vi "Colortable-set.vi"(7 "Invert":bool, 10 "Color table in":dbl[](array[numeric]), 11 "Select CTable 2":T1 items=["blue color", "infrared color", "RB black", "Unchanged", "Purple", "Yellow", "Green", "Red", "'B-W LINEAR'", " 'BLUE-WHITE'", "'GRN-RED-BLU-WHT'", "'RED TEMPERATURE'", "'BLUE-GREEN-RED-YELLOW'", "'STD GAMMA-II'", "'PRISM'", "'RED-PURPLE'", "'GREEN-WHITE LINEAR'", "'GRN-WHT EXPONENTIAL'", "'GREEN-PINK'", "'BLUE-RED'", "'16 LEVEL'", "'RAINBOW'", "'STEPS'", "'STERN SPECIAL'", "'Haze'", "'Blue - Pastel - Red'", "'Pastels'", "'Hue Sat Lightness 1'", "'Hue Sat Lightness 2'", "'Hue Sat Value 1'", "'Hue Sat Value 2'", "'Purple-Red + Stripes'", "'Beach'", "'Mac Style'", "'Eos A'", "'Eos B'", "'Hardcandy'", "'Nature'", "'Ocean'", "'Peppermint'", "'Plasma'", "'Blue-Red'", "'Rainbow'", "'Blue Waves'", "'Volcano'", "'Waves'", "'Rainbow18'", "'Rainbow + white'", "'Rainbow + black'", "'CB-Accent'", "'CB-Dark2'", "'CB-Paired'", "'CB-Pastel1'", "'CB-Pastel2'", "'CB-Set1'", "'CB-Set2'", "'CB-Set3'", "'CB-Blues'", "'CB-BuGn'", "'CB-BuPu'", "'CB-GnBu'", "'CB-Greens'", "'CB-Greys'", "'CB-Oranges'", "'CB-OrRd'", "'CB-PuBu'", "'CB-PuBuGn'", "'CB-PuRd'", "'CB-Purples'", "'CB-RdPu'", "'CB-Reds'", "'CB-YlGn'", "'CB-YlGnBu'", "'CB-YlOrBr'", "'CB-BrBG'", "'CB-PiYG'", "'CB-PRGn'", "'CB-PuOr'", "'CB-RdBu'", "'CB-RdGy'", "'CB-RdYlBu'", "'CB-RdYlG'", "'CB-Spectra'"]) -> (3 "Color table out":u32[](array[numeric]))   [LabVIEW 2019]
uses:
  <userlib>/_Color/Color Table .ctl
panel:
  out "CT index 2":i32 format="%.0x"
  in  "Color Box":u32(colorbox)
  out "CT index":i32
  out "size(s) 2":i32[](array[numeric])
  out "CT name":string
  out "Color tables all 2":u32[][](array[colorbox])
  out "Strings []":string[](array[string])=["blue color", "infrared color", "weird c-table", "Unchanged", "Yellowish", "Green", "Yellow", "B/W", "'B-W LINEAR'", " 'BLUE-WHITE'", "'GRN-RED-BLU-WHT'", "'RED TEMPERATURE'", "'BLUE-GREEN-RED-YELLOW'", "'STD GAMMA-II'", "'PRISM'", "'RED-PURPLE'", "'GREEN-WHITE LINEAR'", "'GRN-WHT EXPONENTIAL'", "'GREEN-PINK'", "'BLUE-RED'", "'16 LEVEL'", "'RAINBOW'", "'STEPS'", "'STERN SPECIAL'", "'Haze'", "'Blue - Pastel - Red'", "'Pastels'", "'Hue Sat Lightness 1'", "'Hue Sat Lightness 2'", "'Hue Sat Value 1'", "'Hue Sat Value 2'", "'Purple-Red + Stripes'", "'Beach'", "'Mac Style'", "'Eos A'", "'Eos B'", "'Hardcandy'", "'Nature'", "'Ocean'", "'Peppermint'", "'Plasma'", "'Blue-Red'", "'Rainbow'", "'Blue Waves'", "'Volcano'", "'Waves'", "'Rainbow18'", "'Rainbow + white'", "'Rainbow + black'", "'CB-Accent'", "'CB-Dark2'", "'CB-Paired'", "'CB-Pastel1'", "'CB-Pastel2'", "'CB-Set1'", "'CB-Set2'", "'CB-Set3'", "'CB-Blues'", "'CB-BuGn'", "'CB-BuPu'", "'CB-GnBu'", "'CB-Greens'", "'CB-Greys'", "'CB-Oranges'", "'CB-OrRd'", "'CB-PuBu'", "'CB-PuBuGn'", "'CB-PuRd'", "'CB-Purples'", "'CB-RdPu'", "'CB-Reds'", "'CB-YlGn'", "'CB-YlGnBu'", "'CB-YlOrBr'", "'CB-BrBG'", "'CB-PiYG'", "'CB-PRGn'", "'CB-PuOr'", "'CB-RdBu'", "'CB-RdGy'", "'CB-RdYlBu'", "'CB-RdYlG'", "'CB-Spectra'"]
  in  "Color tables all":u32[][](array[colorbox])=array75x256[19200 elements]
  in  "color table names":string[](array[string])=["'B-W LINEAR'", " 'BLUE-WHITE'", "'GRN-RED-BLU-WHT'", "'RED TEMPERATURE'", "'BLUE-GREEN-RED-YELLOW'", "'STD GAMMA-II'", "'PRISM'", "'RED-PURPLE'", "'GREEN-WHITE LINEAR'", "'GRN-WHT EXPONENTIAL'", "'GREEN-PINK'", "'BLUE-RED'", "'16 LEVEL'", "'RAINBOW'", "'STEPS'", "'STERN SPECIAL'", "'Haze'", "'Blue - Pastel - Red'", "'Pastels'", "'Hue Sat Lightness 1'", "'Hue Sat Lightness 2'", "'Hue Sat Value 1'", "'Hue Sat Value 2'", "'Purple-Red + Stripes'", "'Beach'", "'Mac Style'", "'Eos A'", "'Eos B'", "'Hardcandy'", "'Nature'", "'Ocean'", "'Peppermint'", "'Plasma'", "'Blue-Red'", "'Rainbow'", "'Blue Waves'", "'Volcano'", "'Waves'", "'Rainbow18'", "'Rainbow + white'", "'Rainbow + black'", "'CB-Accent'", "'CB-Dark2'", "'CB-Paired'", "'CB-Pastel1'", "'CB-Pastel2'", "'CB-Set1'", "'CB-Set2'", "'CB-Set3'", "'CB-Blues'", "'CB-BuGn'", "'CB-BuPu'", "'CB-GnBu'", "'CB-Greens'", "'CB-Greys'", "'CB-Oranges'", "'CB-OrRd'", "'CB-PuBu'", "'CB-PuBuGn'", "'CB-PuRd'", "'CB-Purples'", "'CB-RdPu'", "'CB-Reds'", "'CB-YlGn'", "'CB-YlGnBu'", "'CB-YlOrBr'", "'CB-BrBG'", "'CB-PiYG'", "'CB-PRGn'", "'CB-PuOr'", "'CB-RdBu'", "'CB-RdGy'", "'CB-RdYlBu'", "'CB-RdYlG'", "'CB-Spectra'"]
  out "size(s)":i32
  out "CT array":u32[](array[colorbox])
  out "Color table out 2":dbl[](array[numeric])
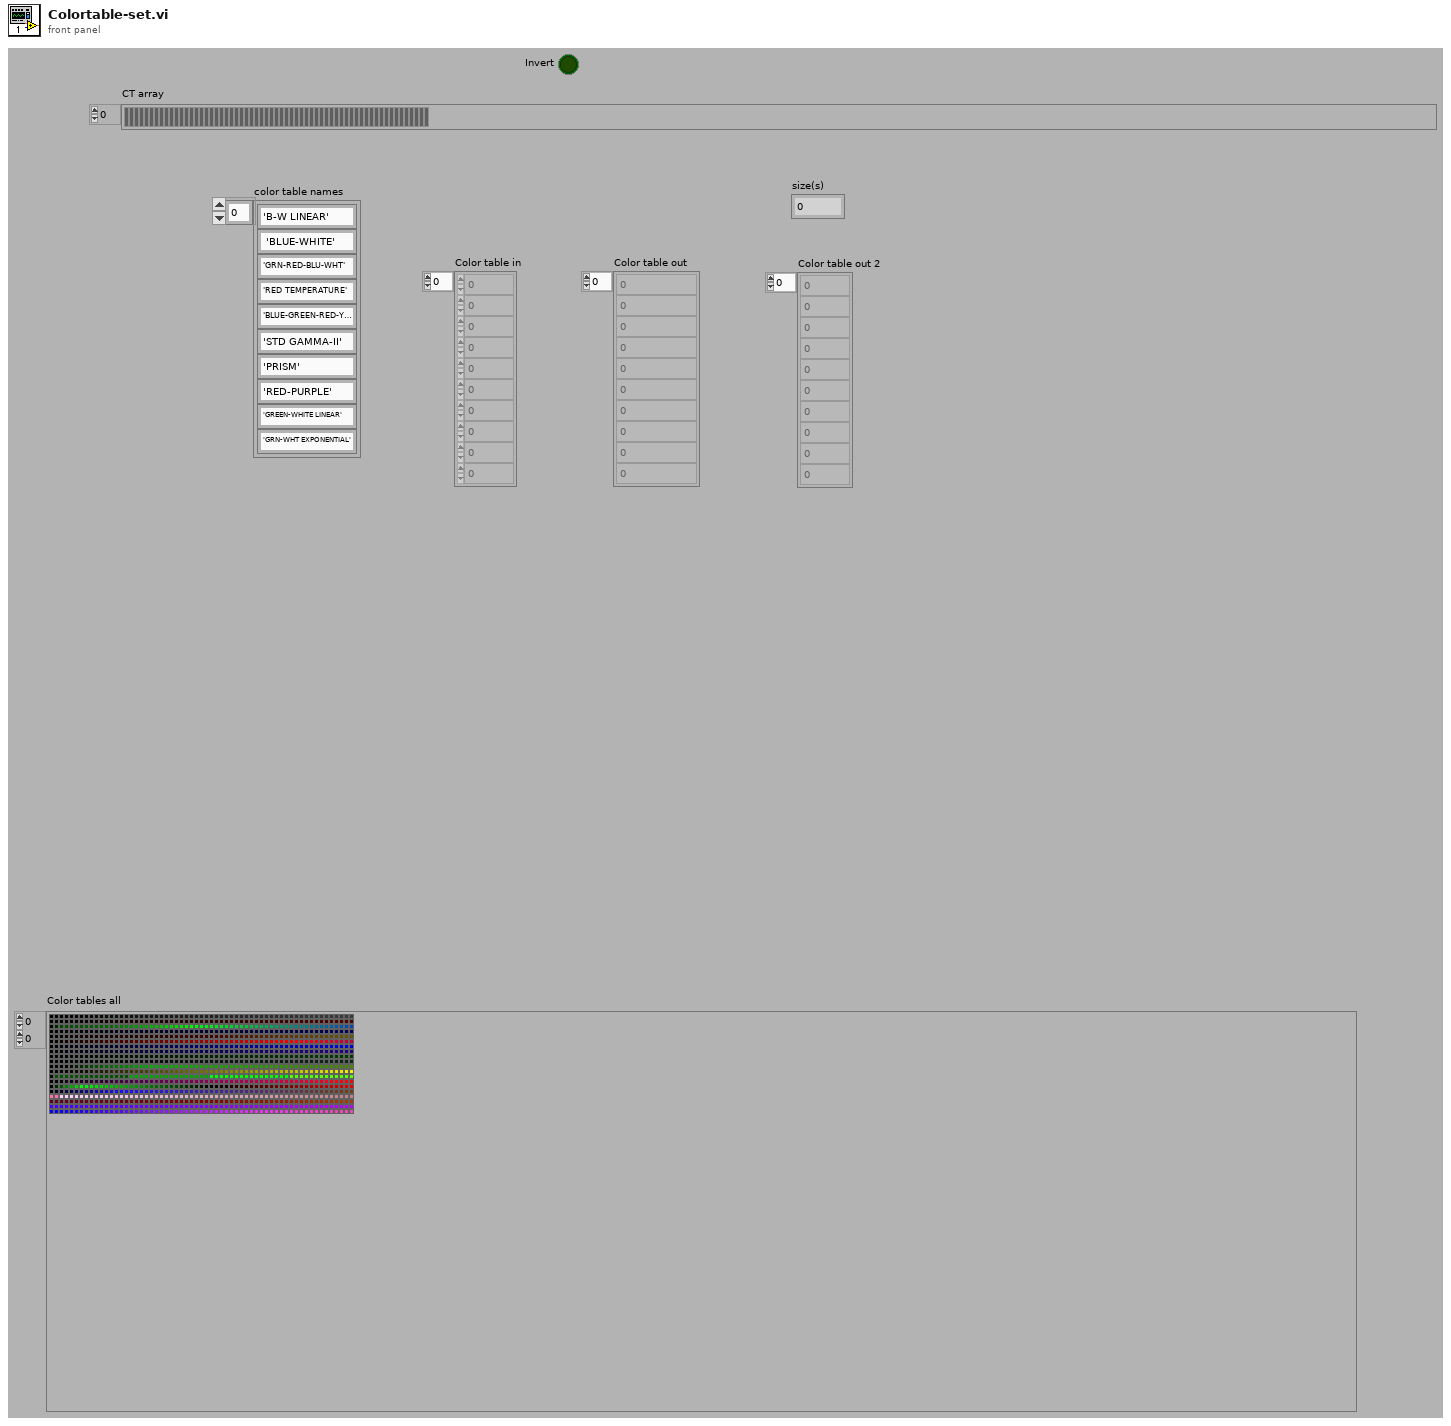
[diagram p1: front panel]
types:
  T1 = typedef "Color Table .ctl" = u16
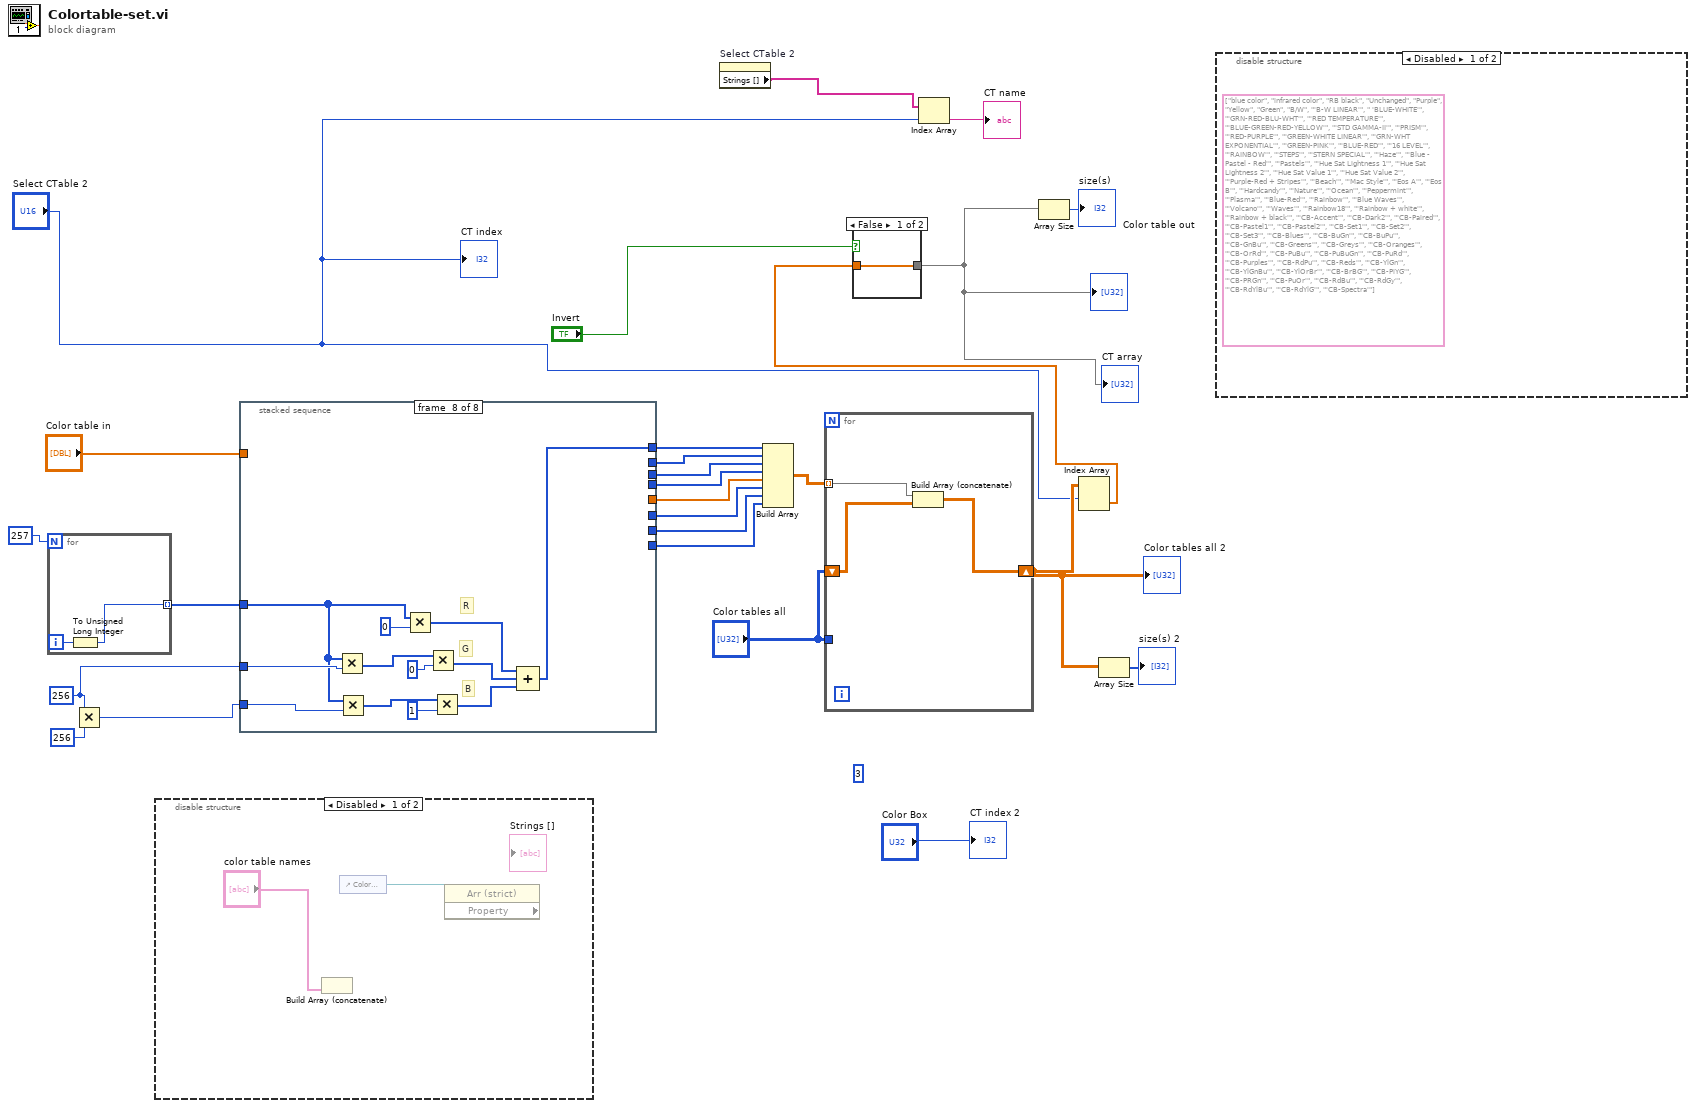
[diagram p0: block diagram]
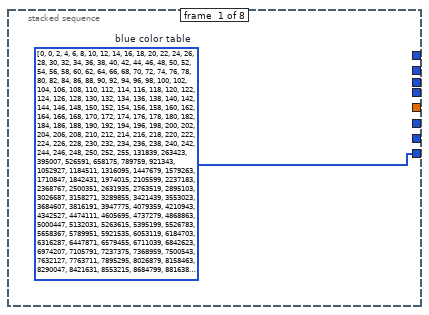
[diagram p3: hidden frame]
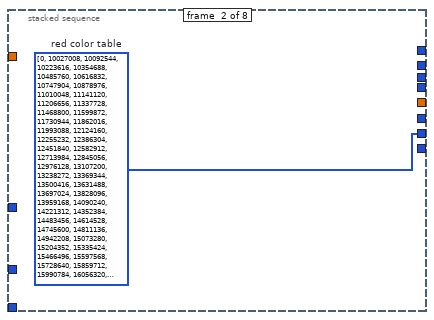
[diagram p4: hidden frame]
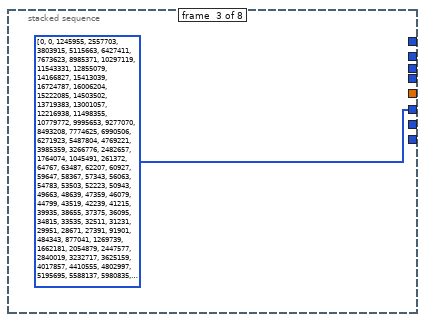
[diagram p5: hidden frame]
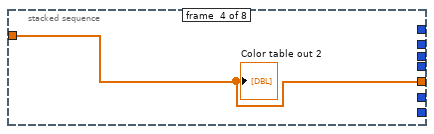
[diagram p6: hidden frame]
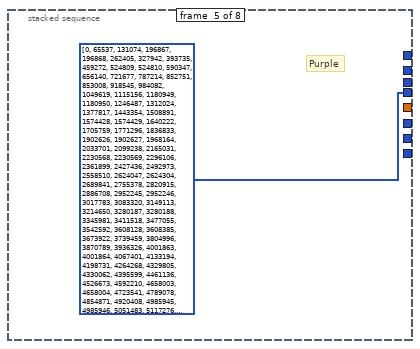
[diagram p7: hidden frame]
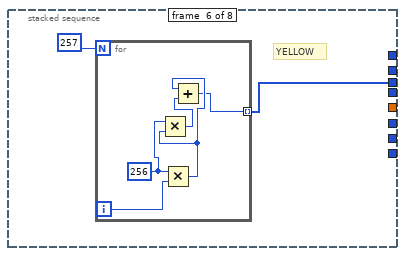
[diagram p8: hidden frame]
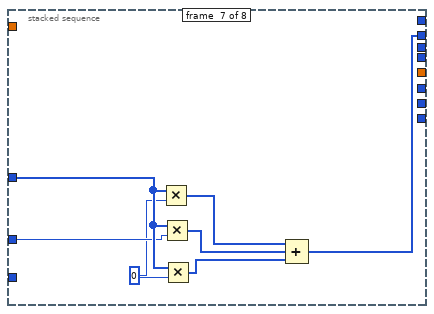
[diagram p9: hidden frame]
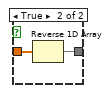
[diagram p11: hidden frame]
diagram:
  w5 = u32 256 ("x")
  (unwired) 3
  n1 = for {
    N: u32 257 -> [_]
    tunnel: [w27] -> w7 mode=indexing
    i -> [w28]
    n2 = To Unsigned Long Integer(number=w28) -> (unsigned 32bit integer=w27:u32)
  }
  n3 = Multiply(x=w5, y=u32 256 ("x")) -> (x*y=w4:u32)
  n4 = disable-structure shown="Disabled" {
    frame Disabled {
      n5 = Build Array (concatenate)("color table names") -> (w31:string[], w32:string[])
      n6 = control-ref of="Color table in"() -> (w30:refnum<vi>)
      n7 = property class="Arr (strict)" props=[](reference=w30) -> ()  [unwired: 1 in, 3 out]
    }
    frame Enabled {
    }
  }
  n8 = stacked-sequence {
    tunnel: "Color table in" -> [_ _ _ w37 _ _ _ _]
    tunnel: [_ _ _ _ u32[] [0, 65537, 131074, 196867, 196868, 262405, 327942, 393735, 459272, 524809, 524810, 590347, 656140, 721677, 787214, 852751, 853008, 918545, 984082, 1049619, 1115156, 1180949, 1180950, 1246487, 1312024, 1377817, 1443354, 1508891, 1574428, 1574429, 1640222, 1705759, 1771296, 1836833, 1902626, 1902627, 1968164, 2033701, 2099238, 2165031, 2230568, 2230569, 2296106, 2361899, 2427436, 2492973, 2558510, 2624047, 2624304, 2689841, 2755378, 2820915, 2886708, 2952245, 2952246, 3017783, 3083320, 3149113, 3214650, 3280187, 3280188, 3345981, 3411518, 3477055, 3542592, 3608128, 3608385, 3673922, 3739459, 3804996, 3870789, 3936326, 4001863, 4001864, 4067401, 4133194, 4198731, 4264268, 4329805, 4330062, 4395599, 4461136, 4526673, 4592210, 4658003, 4658004, 4723541, 4789078, 4854871, 4920408, 4985945, 4985946, 5051483, 5117276, 5182813, 5248350, 5313887, 5379680, 5379681, 5445218, 5510755, 5576292, 5642085, 5707622, 5707623, 5773160, 5838953, 5904490, 5970027, 6035564, 6035565, 6101358, 6166895, 6232432, 6297969, 6363762, 6363763, 6429300, 6494837, 6560374, 6626167, 6691704, 6757241, 6757242, 6823035, 6888572, 6954109, 7019646, 7085183, 7085440, 7150977, 7216514, 7282051, 7347588, 7413381, 7413382, 7478919, 7544456, 7610249, 7675786, 7741323, 7806860, 7806861, 7872654, 7938191, 8003728, 8069265, 8135058, 8135059, 8200596, 8266133, 8331670, 8397463, 8463000, 8463001, 8528538, 8594331, 8659868, 8725405, 8790942, 8790943, 8856736, 8922273, 8987810, 9053347, 9119140, 9184677, 9184678, 9250215, 9315752, 9381545, 9447082, 9512619, 9512620, 9578413, 9643950, 9709487, 9775024, 9840561, 9840818, 9906355, 9971892, 10037429, 10103222, 10168759, 10168760, 10234297, 10299834, 10365627, 10431164, 10496701, 10562238, 10562495, 10628031, 10693568, 10759105, 10824642, 10890435, 10890436, 10955973, 11021510, 11087303, 11152840, 11218377, 11218378, 11283915, 11349708, 11415245, 11480782, 11546319, 11546576, 11612113, 11677650, 11743187, 11808724, 11874517, 11940054, 11940055, 12005592, 12071385, 12136922, 12202459, 12267996, 12267997, 12333790, 12399327, 12464864, 12530401, 12596194, 12596195, 12661732, 12727269, 12792806, 12858599, 12924136, 12989673, 12989674, 13055467, 13121004, 13186541, 13252078, 13317615, 13317872, 13383409, 13448946, 13514483, 13580276, 13645813, 13645814, 13711351, 13776888, 13842681, 13908218, 13973755, 13973756, 14039549, 14105086] ("Clrtbl out") _ _ _] -> w22
    tunnel: [_ _ _ w37 _ _ _ _] -> w21
    tunnel: [_ _ u32[] [0, 0, 1245955, 2557703, 3803915, 5115663, 6427411, 7673623, 8985371, 10297119, 11543331, 12855079, 14166827, 15413039, 16724787, 16006204, 15222085, 14503502, 13719383, 13001057, 12216938, 11498355, 10779772, 9995653, 9277070, 8493208, 7774625, 6990506, 6271923, 5487804, 4769221, 3985359, 3266776, 2482657, 1764074, 1045491, 261372, 64767, 63487, 62207, 60927, 59647, 58367, 57343, 56063, 54783, 53503, 52223, 50943, 49663, 48639, 47359, 46079, 44799, 43519, 42239, 41215, 39935, 38655, 37375, 36095, 34815, 33535, 32511, 31231, 29951, 28671, 27391, 91901, 484343, 877041, 1269739, 1662181, 2054879, 2447577, 2840019, 3232717, 3625159, 4017857, 4410555, 4802997, 5195695, 5588137, 5980835, 6373533, 6765975, 7158673, 7551115, 7943813, 8336511, 8728953, 9121651, 9514093, 9906791, 10299489, 10626396, 11019094, 11411792, 11804234, 12196932, 12589374, 12982072, 13374770, 13767212, 14159910, 14552352, 14945050, 15337748, 15730190, 16122888, 16515330, 16712192, 16713216, 16713984, 16715008, 16716032, 16717056, 16718080, 16718848, 16719872, 16720896, 16721920, 16722944, 16723712, 16724736, 16725760, 16726784, 16727808, 16728576, 16729600, 16730624, 16731648, 16732672, 16733440, 16734464, 16735488, 16736512, 16737280, 16738304, 16739328, 16740352, 16741376, 16742144, 16743168, 16744192, 16745216, 16746240, 16747008, 16748032, 16749056, 16750080, 16751104, 16751872, 16752896, 16753920, 16754944, 16755968, 16756736, 16757760, 16758784, 16759808, 16760832, 16761600, 16762624, 16763648, 16370944, 15912448, 15454208, 14995712, 14471936, 14013440, 13554944, 13096704, 12572672, 12114432, 11655936, 11197696, 10739200, 10215424, 9756928, 9298432, 8840192, 8316160, 7857920, 7399424, 6941184, 6417152, 5958912, 5500416, 5041920, 4518144, 4059648, 3601408, 3142912, 2619136, 2160640, 1702400, 1243904, 720128, 261632, 261890, 589574, 982794, 1310478, 1703699, 2031383, 2424603, 2752287, 3145507, 3473191, 3866411, 4194095, 4587316, 4915000, 5308220, 5635904, 6029124, 6356808, 6750028, 7077712, 7470933, 7798617, 8191837, 8519521, 8912741, 9240425, 9633645, 9961329, 10354550, 10682234, 11075454, 11403138, 11796358, 12124042, 12517262, 12844946, 13238167, 13434777, 13434777, 13434777, 13434777, 13434777, 13434777, 13434777, 13434777, 13434777, 13434777, 13434777, 13434777, 13434777, 13434777, 13434777, 13434777, 13434777, 13434777, 16777215] ("Write Attribute") _ _ _ _ _] -> w20
    tunnel: [_ w35 _ _ _ _ _ _] -> w19
    tunnel: [w34 _ _ _ _ _ _ _] -> w18
    tunnel: [_ _ _ _ _ w39 _ _] -> w11
    tunnel: [_ _ _ _ _ _ w50 _] -> w10
    tunnel: w7 -> [_ _ _ _ _ _ w49 w59]
    tunnel: w5 -> [_ _ _ _ _ _ w47 w61]
    tunnel: w4 -> [_ _ _ _ _ _ _ w60]
    tunnel: [_ _ _ _ _ _ _ w62] -> w1
    frame #0 {
      w34 = u32[] [0, 0, 2, 4, 6, 8, 10, 12, 14, 16, 18, 20, 22, 24, 26, 28, 30, 32, 34, 36, 38, 40, 42, 44, 46, 48, 50, 52, 54, 56, 58, 60, 62, 64, 66, 68, 70, 72, 74, 76, 78, 80, 82, 84, 86, 88, 90, 92, 94, 96, 98, 100, 102, 104, 106, 108, 110, 112, 114, 116, 118, 120, 122, 124, 126, 128, 130, 132, 134, 136, 138, 140, 142, 144, 146, 148, 150, 152, 154, 156, 158, 160, 162, 164, 166, 168, 170, 172, 174, 176, 178, 180, 182, 184, 186, 188, 190, 192, 194, 196, 198, 200, 202, 204, 206, 208, 210, 212, 214, 216, 218, 220, 222, 224, 226, 228, 230, 232, 234, 236, 238, 240, 242, 244, 246, 248, 250, 252, 255, 131839, 263423, 395007, 526591, 658175, 789759, 921343, 1052927, 1184511, 1316095, 1447679, 1579263, 1710847, 1842431, 1974015, 2105599, 2237183, 2368767, 2500351, 2631935, 2763519, 2895103, 3026687, 3158271, 3289855, 3421439, 3553023, 3684607, 3816191, 3947775, 4079359, 4210943, 4342527, 4474111, 4605695, 4737279, 4868863, 5000447, 5132031, 5263615, 5395199, 5526783, 5658367, 5789951, 5921535, 6053119, 6184703, 6316287, 6447871, 6579455, 6711039, 6842623, 6974207, 7105791, 7237375, 7368959, 7500543, 7632127, 7763711, 7895295, 8026879, 8158463, 8290047, 8421631, 8553215, 8684799, 8816383, 8947967, 9079551, 9211135, 9342719, 9474303, 9605887, 9737471, 9869055, 10000639, 10132223, 10263807, 10395391, 10526975, 10658559, 10790143, 10921727, 11053311, 11184895, 11316479, 11448063, 11579647, 11711231, 11842815, 11974399, 12105983, 12237567, 12369151, 12500735, 12632319, 12763903, 12895487, 13027071, 13158655, 13290239, 13421823, 13553407, 13684991, 13816575, 13948159, 14079743, 14211327, 14342911, 14474495, 14606079, 14737663, 14869247, 15000831, 15132415, 15263999, 15395583, 15527167, 15658751, 15790335, 15921919, 16053503, 16185087, 16316671, 16448255, 16579839, 16777215]  # blue color table
    }
    frame #1 {
      w35 = u32[] [0, 10027008, 10092544, 10223616, 10354688, 10485760, 10616832, 10747904, 10878976, 11010048, 11141120, 11206656, 11337728, 11468800, 11599872, 11730944, 11862016, 11993088, 12124160, 12255232, 12386304, 12451840, 12582912, 12713984, 12845056, 12976128, 13107200, 13238272, 13369344, 13500416, 13631488, 13697024, 13828096, 13959168, 14090240, 14221312, 14352384, 14483456, 14614528, 14745600, 14811136, 14942208, 15073280, 15204352, 15335424, 15466496, 15597568, 15728640, 15859712, 15990784, 16056320, 16187392, 16318464, 16449536, 16580608, 16711680, 16711936, 16711936, 16712192, 16712448, 16712704, 16712960, 16713216, 16713472, 16713472, 16713728, 16713984, 16714240, 16714496, 16714752, 16715008, 16715008, 16715264, 16715520, 16715776, 16716032, 16716288, 16716544, 16716544, 16716800, 16717056, 16717312, 16717568, 16717824, 16718080, 16718080, 16718336, 16718592, 16718848, 16719104, 16719360, 16719616, 16719872, 16719872, 16720128, 16720384, 16720640, 16720896, 16721152, 16721408, 16721408, 16721664, 16721920, 16722176, 16722432, 16722688, 16722944, 16722944, 16723200, 16723456, 16723712, 16723968, 16724224, 16724480, 16724480, 16724736, 16724992, 16724992, 16725248, 16725504, 16725760, 16725760, 16726016, 16726272, 16726272, 16726528, 16726784, 16726784, 16727040, 16727296, 16727296, 16727552, 16727808, 16728064, 16728064, 16728320, 16728576, 16728576, 16728832, 16729088, 16729088, 16729344, 16729600, 16729600, 16729856, 16730112, 16730112, 16730368, 16730624, 16730880, 16730880, 16731136, 16731392, 16731392, 16731648, 16731904, 16731904, 16732160, 16732416, 16732416, 16732672, 16732928, 16732928, 16733184, 16733440, 16733696, 16733696, 16733952, 16734208, 16734208, 16734464, 16734720, 16734720, 16734976, 16735232, 16735232, 16735488, 16735744, 16735744, 16736000, 16736256, 16736512, 16736512, 16736768, 16737024, 16737024, 16737280, 16737536, 16737536, 16738048, 16738560, 16739328, 16739840, 16740352, 16741120, 16741632, 16742144, 16742912, 16743424, 16743936, 16744448, 16745216, 16745728, 16746240, 16747008, 16747520, 16748032, 16748544, 16749312, 16749824, 16750336, 16751104, 16751616, 16752128, 16752896, 16753408, 16753920, 16754432, 16755200, 16755712, 16756224, 16756992, 16757504, 16758016, 16758528, 16759296, 16759808, 16760320, 16761088, 16761600, 16762112, 16762624, 16763392, 16763904, 16764416, 16765184, 16765696, 16766208, 16766976, 16767488, 16768000, 16768512, 16769280, 16769792, 16770304, 16771072, 16771584, 16772096, 16772608, 16773376, 16773888, 16774400, 16775168, 16775680, 16776192, 16777215]  # red color table
    }
    frame #2 {
    }
    frame #3 {
      "Color table out 2" <- w37
    }
    frame #4 {
      # "Purple"
    }
    frame #5 {
      # "YELLOW"
      n9 = for {
        N: 257 -> [_]
        tunnel: [w41] -> w39 mode=indexing
        i -> [w45]
        w44 = 256 ("x")
        n10 = Multiply(x=w44, y=w45) -> (x*y=w42:i32)
        n11 = Multiply(x=w44, y=w42) -> (x*y=w43:i32)
        n12 = Add(x=w42, y=w43) -> (x+y=w41:i32)
      }
    }
    frame #6 {
      w46 = 0
      n13 = Multiply(x=w49, y=w46) -> (x*y=w48:u32[])
      n14 = Multiply(x=w49, y=w47) -> (x*y=w52:u32[])
      n15 = Multiply(x=w49, y=w46) -> (x*y=w51:u32[])
      n16 = Compound Arithmetic op=ADD(w48, w52, w51) -> (w50:u32[])
    }
    frame #7 {
      # "B"
      # "G"
      # "R"
      n17 = Multiply(x=w59, y=w61) -> (x*y=w55:u32[])
      n18 = Multiply(x=w59, y=w60) -> (x*y=w64:u32[])
      n19 = Multiply(x=w59, y=0) -> (x*y=w63:u32[])
      n20 = Multiply(x=w55, y=0) -> (x*y=w57:u32[])
      n21 = Multiply(x=w64, y=1) -> (x*y=w56:u32[])
      n22 = Compound Arithmetic op=ADD(w63, w57, w56) -> (w62:u32[])
    }
  }
  n23 = property on="Select CTable 2" class="Ring (strict)"() -> ("Strings []"=w2:string[])  [unwired: 2 in, 2 out]
  n24 = Build Array(w1, w10, w11, w22, w21, w20, w19, w18) -> (w15:dbl[][])
  n25 = for {
    tunnel: "Color tables all" -> [_]
    tunnel: w15 -> [w65] mode=indexing
    shift-right: [w67] -> w13
    shift-left: "Color tables all" -> [w66]
    n26 = Build Array (concatenate)(w65, w66) -> (w67:dbl[][])
  }
  "Color tables all 2" <- w13
  n27 = Index Array(array=w2, index="Select CTable 2") -> (element=→"CT name":string)
  n28 = Index Array(array=w13, index (row)="Select CTable 2") -> (element=w16:dbl[])  [unwired: 1 in]
  n29 = case shown="False" "Invert" {
    tunnel: w16 -> [w68 w70]
    tunnel: [w68 w69] -> w25
    frame False {
    }
    frame True {
      n30 = Reverse 1D Array(array=w70) -> (reversed array=w69:dbl[])
    }
  }
  "Color table out" <- w25
  "CT array" <- w25
  n31 = Array Size(array=w25) -> (size(s)=→"size(s)":i32)
  n32 = Array Size(array=w13) -> (size(s)=→"size(s) 2":i32[])
  n33 = disable-structure shown="Disabled" {
    frame Disabled {
      w71 = string[] ["blue color", "infrared color", "RB black", "Unchanged", "Purple", "Yellow", "Green", "B/W", "'B-W LINEAR'", " 'BLUE-WHITE'", "'GRN-RED-BLU-WHT'", "'RED TEMPERATURE'", "'BLUE-GREEN-RED-YELLOW'", "'STD GAMMA-II'", "'PRISM'", "'RED-PURPLE'", "'GREEN-WHITE LINEAR'", "'GRN-WHT EXPONENTIAL'", "'GREEN-PINK'", "'BLUE-RED'", "'16 LEVEL'", "'RAINBOW'", "'STEPS'", "'STERN SPECIAL'", "'Haze'", "'Blue - Pastel - Red'", "'Pastels'", "'Hue Sat Lightness 1'", "'Hue Sat Lightness 2'", "'Hue Sat Value 1'", "'Hue Sat Value 2'", "'Purple-Red + Stripes'", "'Beach'", "'Mac Style'", "'Eos A'", "'Eos B'", "'Hardcandy'", "'Nature'", "'Ocean'", "'Peppermint'", "'Plasma'", "'Blue-Red'", "'Rainbow'", "'Blue Waves'", "'Volcano'", "'Waves'", "'Rainbow18'", "'Rainbow + white'", "'Rainbow + black'", "'CB-Accent'", "'CB-Dark2'", "'CB-Paired'", "'CB-Pastel1'", "'CB-Pastel2'", "'CB-Set1'", "'CB-Set2'", "'CB-Set3'", "'CB-Blues'", "'CB-BuGn'", "'CB-BuPu'", "'CB-GnBu'", "'CB-Greens'", "'CB-Greys'", "'CB-Oranges'", "'CB-OrRd'", "'CB-PuBu'", "'CB-PuBuGn'", "'CB-PuRd'", "'CB-Purples'", "'CB-RdPu'", "'CB-Reds'", "'CB-YlGn'", "'CB-YlGnBu'", "'CB-YlOrBr'", "'CB-BrBG'", "'CB-PiYG'", "'CB-PRGn'", "'CB-PuOr'", "'CB-RdBu'", "'CB-RdGy'", "'CB-RdYlBu'", "'CB-RdYlG'", "'CB-Spectra'"]
    }
    frame Enabled {
    }
  }
  "CT index" <- "Select CTable 2"
  "CT index 2" <- "Color Box"
